vi "Register for Camera Events.vi"(8 "error in (no error)":errorcluster, 11 "Camera Async Coms in":refnum<class "Camera Async Coms.lvclass">) -> (0 "error out":errorcluster, 2 "output cluster":T1, 3 "Camera Async Coms out":refnum<class "Camera Async Coms.lvclass">)   [LabVIEW 2022 SP3, in "Camera Async Coms.lvclass"]
uses:
  Camera Async Coms.lvclass
  <vilib>/vision/Image Controls.llb/IMAQ Image.ctl
  Camera Data/events.ctl
  Camera Data/Camera Data.lvclass
  XY Stage/Process Actor/Process Framework/Process State Data/Events.ctl
  XY Stage/Process Actor/Process Framework/Process State Data/Process State Data.lvclass
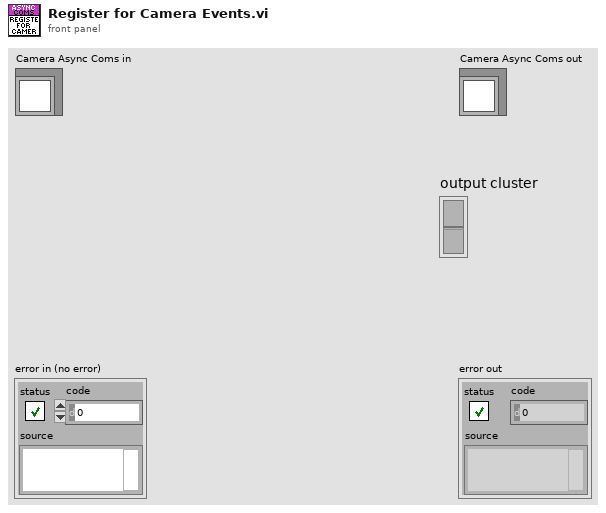
[diagram p1: front panel]
types:
  T1 = cluster{"Event Registration Refnum":refnum<event-registration>, "Event Registration Refnum":refnum<event-registration>}
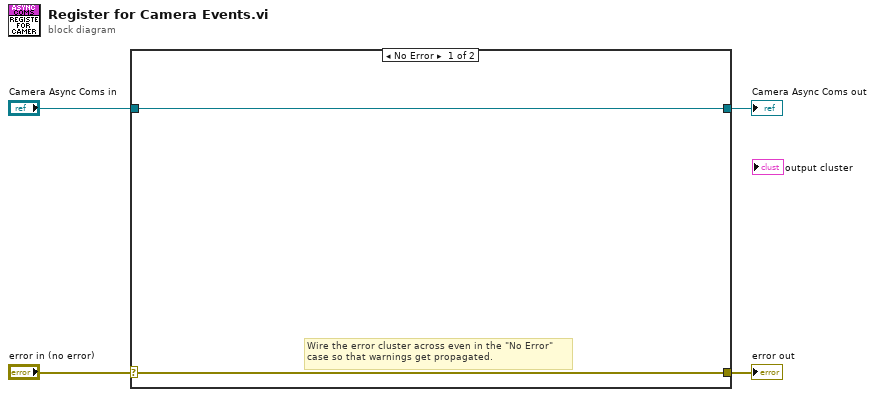
[diagram p0: block diagram]
diagram:
  n1 = case shown="No Error" "error in (no error)" {
    selector: "error in (no error)" -> [w5 w8]
    tunnel: [w5 w8] -> w3
    tunnel: [w6 w7] -> w1
    tunnel: "Camera Async Coms in" -> [w6 w7]
    frame No Error {
      # "Wire the error cluster across even in the \"No Error\"\ncase so that warnings get propagated."
    }
    frame Error {
    }
  }
  "error out" <- w3
  "Camera Async Coms out" <- w1
